vi "Varian Magnet Control Panel (No Objects).vi"(8 "error in":errorcluster) -> (0 "error out":errorcluster)   [LabVIEW 2012]
panel:
  in  "Maintain Field":bool
  in  "Time per Point (ms)":i32=100
  out "Waveform Chart":dbl[unit](graph)
  in  "Read current field":bool
  in  "Go to field (immediately)":bool
  out "Current Field":dbl[unit]
  in  "Desired field":dbl[unit]
  in  "stop":bool
  # "Min Field ~0.03T"
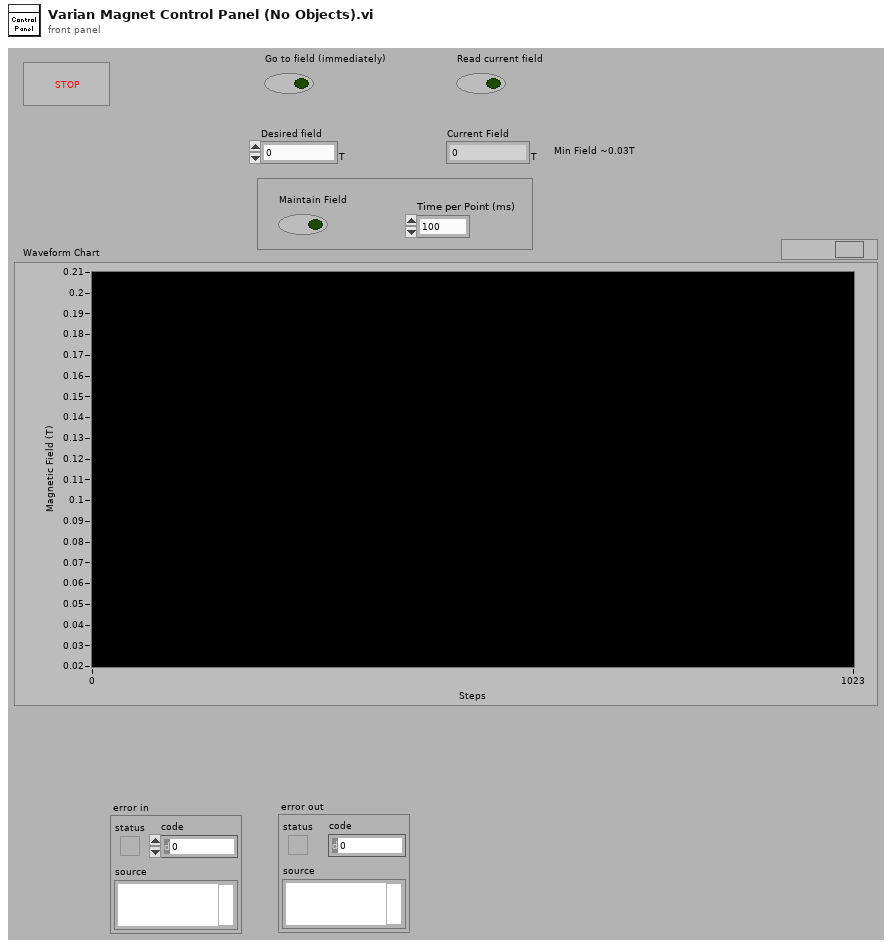
[diagram p1: front panel]
types:
  T1 = cluster{"Fluke VISA resource name":refnum<visa-resource-name>, "DAQ Physical Channel":tag, "DAQ Task - Set":refnum<k21>, "DAQ Task - Read":refnum<k21>, "Control Voltage":enum16{"Please Select a Value", "30V", "40V"}, "extrapolated":cluster{"x locations":dbl[], "coefficients":dbl[][]}, "last 5 field numbers":dbl[], "Fluke Multimeter":cluster{"function (0:volts DC)":u16, "range (0:auto)":u16, "rate (0:slow)":u16, "trigger mode (0:internal)":u16, "Autorange":bool}}
  T2 = typedef "NI_Gmath.lvlib/in_piecewise interp poly control.ctl" = cluster{"x locations":dbl[], "coefficients":dbl[][]}
  T3 = cluster{"Fluke VISA resource name":refnum<visa-resource-name>, "DAQ Physical Channel":tag, "DAQ Task - Set":refnum<k21>, "DAQ Task - Read":refnum<k21>, "Control Voltage":enum16{"Please Select a Value", "30V", "40V"}, "extrapolated":T2, "last 5 field numbers":dbl[], "Fluke Multimeter":cluster{"function (0:volts DC)":u16, "range (0:auto)":u16, "rate (0:slow)":u16, "trigger mode (0:internal)":u16, "Autorange":bool}}
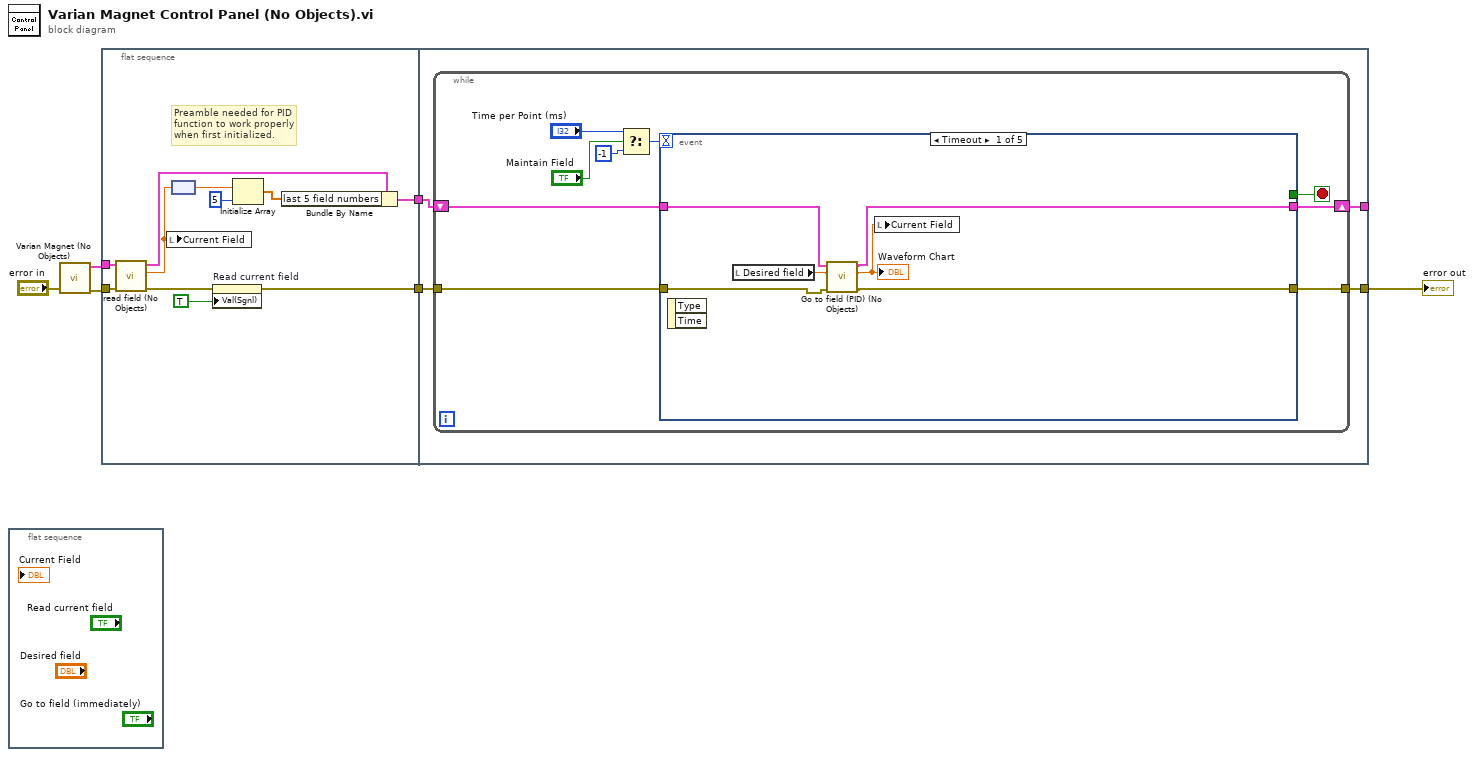
[diagram p0: block diagram]
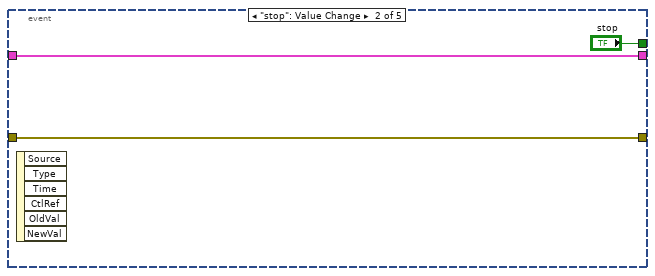
[diagram p2: hidden frame]
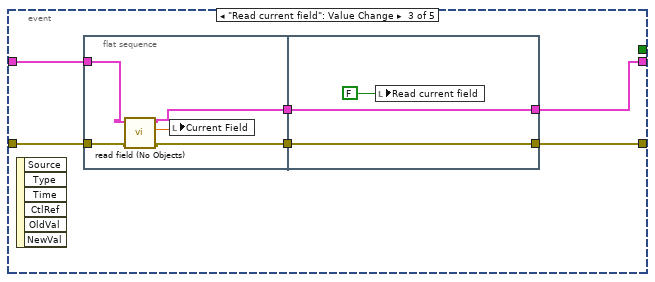
[diagram p3: hidden frame]
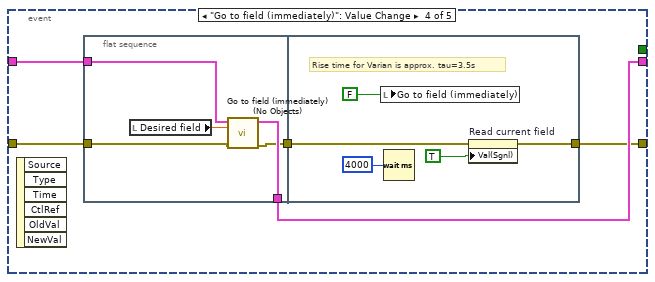
[diagram p4: hidden frame]
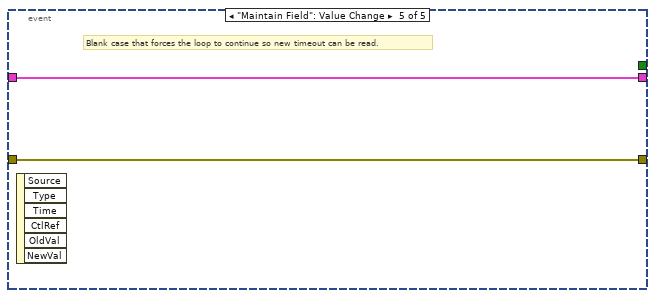
[diagram p5: hidden frame]
diagram:
  n1 = flat-sequence {
    frame #0 {
    }
  }
  n2 = call "Varian Magnet (No Objects).vi"("error in (no error)"="error in") -> ("error out"=w2:errorcluster, "Varian Magnet out"=w1:T1)  [unwired: 9 in]
  n3 = flat-sequence {
    tunnel: [w15] -> w6
    tunnel: [w13] -> w5
    tunnel: w1 -> [w9]
    tunnel: w2 -> [w11]
    tunnel: w6 -> [w18]
    tunnel: [w21] -> _
    tunnel: w5 -> [w20]
    tunnel: [w19] -> w4
    frame #0 {
      # "Preamble needed for PID\nfunction to work properly\nwhen first initialized."
      n4 = call "read field (No Objects).vi"("error in (no error)"=w11, "Varian Magnet In"=w9) -> ("error out"=w10:errorcluster, "Field"=w7:dbl[unit], "Varian Magnet Out"=w8:T3)  [unwired: 7 in]
      n5 = local write "Current Field"(w7) -> ()
      n6 = node(w7) -> (w12:dbl)
      n7 = property on="Read current field" class="Bool (strict)"(error in=w10, "Val(Sgnl)"=TRUE ("Value (Signaling)")) -> (error out=w13:errorcluster)  [unwired: 1 in, 1 out]
      n8 = Initialize Array(w12, 5 ("dimension size")) -> (w16:dbl[])
      n9 = Bundle By Name(cluster=w8, "last 5 field numbers"=w16) -> (w15:T3)
    }
    frame #1 {
      n10 = while {
        tunnel: w20 -> [w28]
        tunnel: [w27] -> w19
        shift-right: [w29] -> w21
        shift-left: w18 -> [w26]
        stop <- w30 stop-if-true
        n11 = Select(t="Time per Point (ms)", s="Maintain Field", f=-1) -> (s? t:f=w22:i32)
        n12 = event shown="[0] Timeout" {
          selector: _ -> [_ _ _ _ _]
          dyn-events: _ -> [_ _ _ _ _]
          timeout: w22 -> [_ _ _ _ _]
          tunnel: [_ "stop" _ _ _] -> w30
          tunnel: w26 -> [w34 w38 w43 w57 w70]
          tunnel: [w33 w38 w42 w56 w70] -> w29
          tunnel: w28 -> [w36 w37 w45 w58 w69]
          tunnel: [w35 w37 w44 w54 w69] -> w27
          event Timeout {
            n13 = event-data() -> ()  [unwired: 3 out]
            n14 = local read "Desired field"() -> (w32:dbl[unit])
            n15 = call "Go to field (PID) (No Objects).vi"("error in (no error)"=w36, "Desired Field"=w32, "Varian Magnet In"=w34) -> ("error out"=w35:errorcluster, "Current Field"=w31:dbl[unit], "Varian Magnet Out"=w33:T3)  [unwired: 5 in, 1 out]
            "Waveform Chart" <- w31
            n16 = local write "Current Field"(w31) -> ()
          }
          event "stop": Value Change {
            n17 = event-data() -> ()  [unwired: 7 out]
          }
          event "Read current field": Value Change {
            n18 = event-data() -> ()  [unwired: 7 out]
            n19 = flat-sequence {
              tunnel: w45 -> [w49]
              tunnel: w43 -> [w46]
              tunnel: [w48] -> w41
              tunnel: [w47] -> w40
              tunnel: [w52] -> w42
              tunnel: [w53] -> w44
              tunnel: w41 -> [w53]
              tunnel: w40 -> [w52]
              frame #0 {
                n20 = call "read field (No Objects).vi"("error in (no error)"=w49, "Varian Magnet In"=w46) -> ("error out"=w48:errorcluster, "Field"=w50:dbl[unit], "Varian Magnet Out"=w47:T3)  [unwired: 7 in]
                n21 = local write "Current Field"(w50) -> ()
              }
              frame #1 {
                n22 = local write "Read current field"(FALSE ("Read current field")) -> ()
              }
            }
          }
          event "Go to field (immediately)": Value Change {
            n23 = event-data() -> ()  [unwired: 7 out]
            n24 = flat-sequence {
              tunnel: w58 -> [w62]
              tunnel: w57 -> [w61]
              tunnel: [w60] -> w56
              tunnel: [w59] -> w55
              tunnel: [w66] -> w54
              tunnel: w55 -> [w67]
              frame #0 {
                n25 = local read "Desired field"() -> (w63:dbl[unit])
                n26 = call "Go to field (immediately) (No Objects).vi"("error in"=w62, "Desired field (T)"=w63, "Varian Magnet In"=w61) -> ("error out"=w59:errorcluster, "Varian Magnet Out"=w60:T3)  [unwired: 7 in]
              }
              frame #1 {
                # "Rise time for Varian is approx. tau=3.5s"
                n27 = local write "Go to field (immediately)"(FALSE ("Value (Signaling)")) -> ()
                n28 = Wait (ms)(milliseconds to wait=u32 4000) -> ()  [unwired: 1 out]
                n29 = property on="Read current field" class="Bool (strict)"(error in=w67, "Val(Sgnl)"=TRUE ("Value (Signaling)")) -> (error out=w66:errorcluster)  [unwired: 1 in, 1 out]
              }
            }
          }
          event "Maintain Field": Value Change {
            # "Blank case that forces the loop to continue so new timeout can be read."
            n30 = event-data() -> ()  [unwired: 7 out]
          }
        }
      }
    }
  }
  "error out" <- w4
